vi "Test Master API.vi"() -> ()   [LabVIEW 2021, in "Master.lvlib"]
doc: "Master API Tester.\n\n<b>Note:</b> This VI was modified by the <b>Validate DQMH Module</b> tool to remove code to stop the main loop on error, and instead display the most recent error on the tester front panel."
uses:
  Master.lvlib
  <vilib>/Utility/error.llb/DialogType.ctl
panel:
  out "last error":errorcluster
  in  "SlaveID":i32(ring)=-1 items=["All"=-1, "1"=1, "2"=2, "3"=3, "4"=4, "5"=5, "6"=6, "7"=7, "8"=8, "9"=9, "10"=10, "11"=11, "12"=12, "13"=13, "14"=14, "15"=15, "16"=16, "17"=17, "18"=18, "19"=19, "20"=20, "21"=21, "22"=22, "23"=23, "24"=24, "25"=25, "26"=26, "27"=27, "28"=28, "29"=29, "30"=30, "31"=31, "32"=32, "33"=33, "34"=34, "35"=35, "36"=36, "37"=37, "38"=38, "39"=39, "40"=40, "41"=41, "42"=42, "43"=43, "44"=44, "45"=45, "46"=46, "47"=47, "48"=48, "49"=49, "50"=50, "51"=51, "52"=52, "53"=53, "54"=54, "55"=55, "56"=56, "57"=57, "58"=58, "59"=59, "60"=60, "61"=61, "62"=62, "63"=63, "64"=64, "65"=65, "66"=66, "67"=67, "68"=68, "69"=69, "70"=70, "71"=71, "72"=72, "73"=73, "74"=74, "75"=75, "76"=76, "77"=77, "78"=78, "79"=79, "80"=80, "81"=81, "82"=82, "83"=83, "84"=84, "85"=85, "86"=86, "87"=87, "88"=88, "89"=89, "90"=90, "91"=91, "92"=92, "93"=93, "94"=94, "95"=95, "96"=96, "97"=97, "98"=98, "99"=99, "100"=100, "101"=101, "102"=102, "103"=103, "104"=104, "105"=105, "106"=106, "107"=107, "108"=108, "109"=109, "110"=110, "111"=111, "112"=112, "113"=113, "114"=114, "115"=115, "116"=116, "117"=117, "118"=118, "119"=119, "120"=120, "121"=121, "122"=122, "123"=123, "124"=124, "125"=125, "126"=126, "127"=127, "128"=128, "129"=129, "130"=130, "131"=131, "132"=132, "133"=133, "134"=134, "135"=135, "136"=136, "137"=137, "138"=138, "139"=139, "140"=140, "141"=141, "142"=142, "143"=143, "144"=144, "145"=145, "146"=146, "147"=147, "148"=148, "149"=149, "150"=150, "151"=151, "152"=152, "153"=153, "154"=154, "155"=155, "156"=156, "157"=157, "158"=158, "159"=159, "160"=160, "161"=161, "162"=162, "163"=163, "164"=164, "165"=165, "166"=166, "167"=167, "168"=168, "169"=169, "170"=170, "171"=171, "172"=172, "173"=173, "174"=174, "175"=175, "176"=176, "177"=177, "178"=178, "179"=179, "180"=180, "181"=181, "182"=182]
  in  "Slave Stop":bool
  in  "Slave Launch":bool
  out "Title":string
  in  "Show Diagram on Init":bool
  in  "Show Block Diagram":bool
  in  "Stop Module":bool
  in  "Start Module":bool
  in  "Hide Module Panel":bool
  in  "Show Module Panel":bool
  out "Status":string
  out "Module Running?":bool
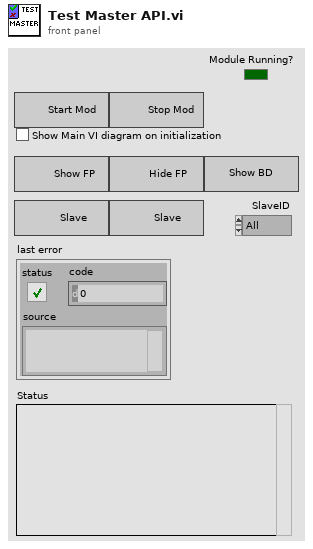
[diagram p1: front panel]
types:
  T1 = typedef "Master.lvlib/Broadcast Events--cluster.ctl" = cluster{"Module Did Init":refnum<user-event>, "Status Updated":refnum<user-event>, "Error Reported":refnum<user-event>, "Module Did Stop":refnum<user-event>, "Update Module Execution Status":refnum<user-event>, "Slave Launched":refnum<user-event>}
  T2 = typedef "DialogType.ctl" = u16
  T3 = typedef "LVStringsAndValuesArrayTypeDef_I32.ctl" = cluster{"String":string, "Value":i32}[]
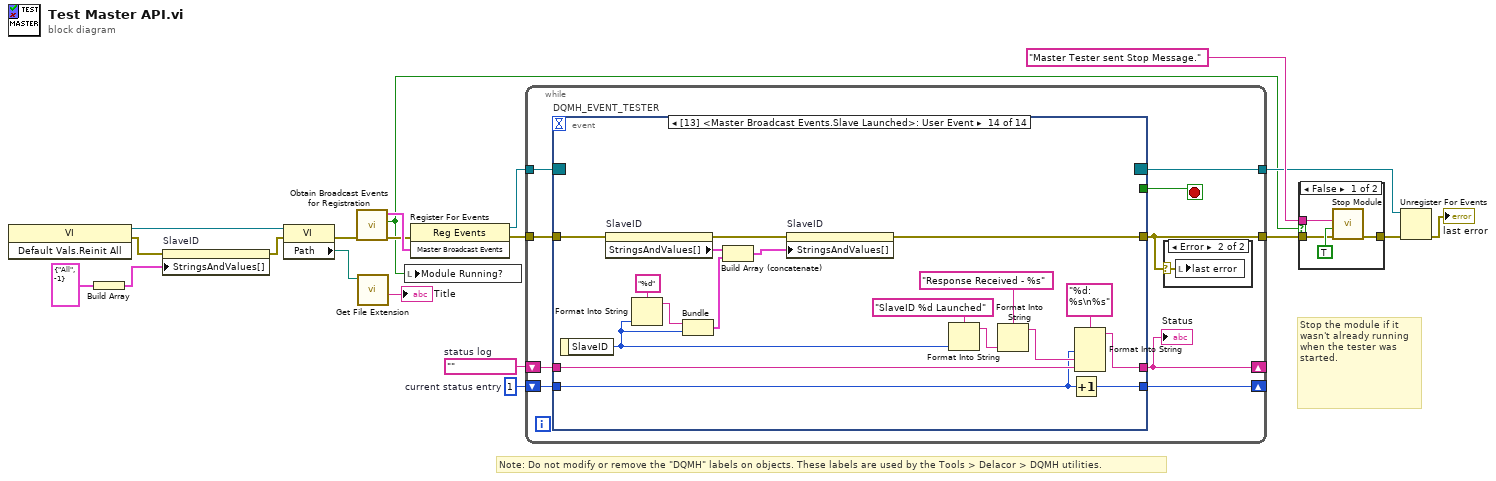
[diagram p0: block diagram]
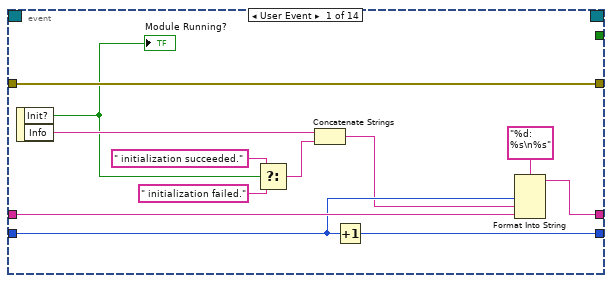
[diagram p4: hidden frame]
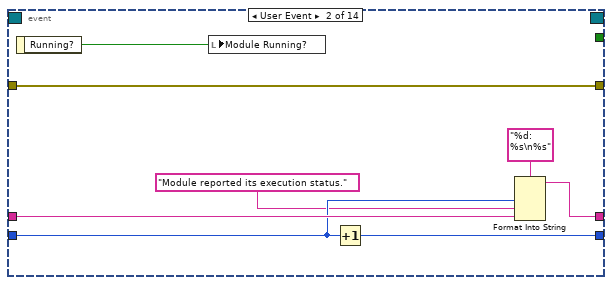
[diagram p5: hidden frame]
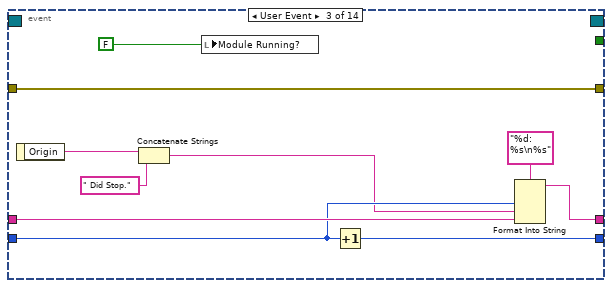
[diagram p6: hidden frame]
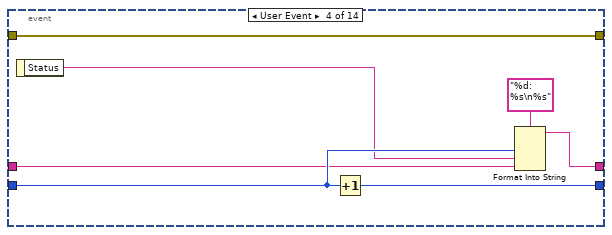
[diagram p7: hidden frame]
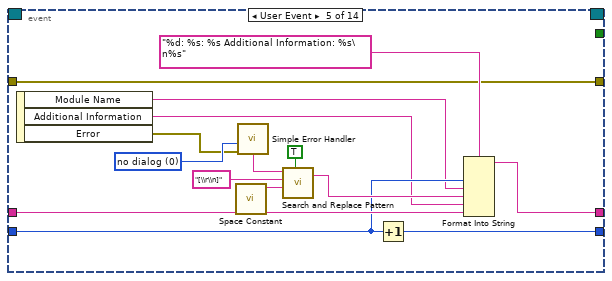
[diagram p8: hidden frame]
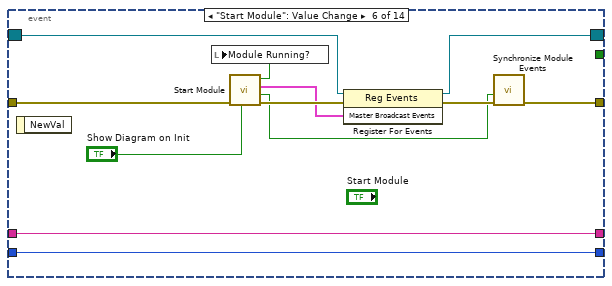
[diagram p9: hidden frame]
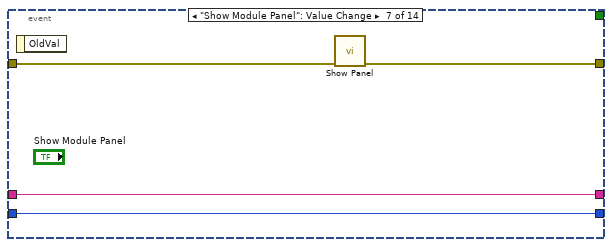
[diagram p10: hidden frame]
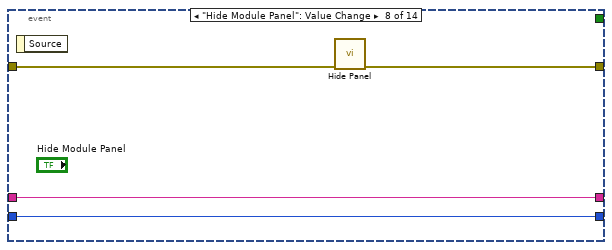
[diagram p11: hidden frame]
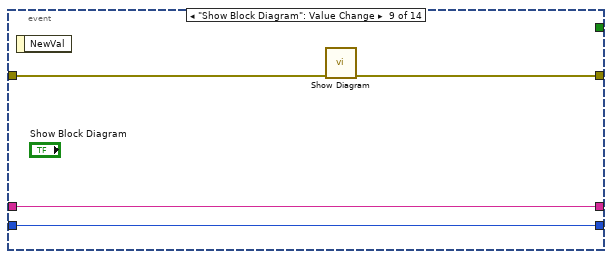
[diagram p12: hidden frame]
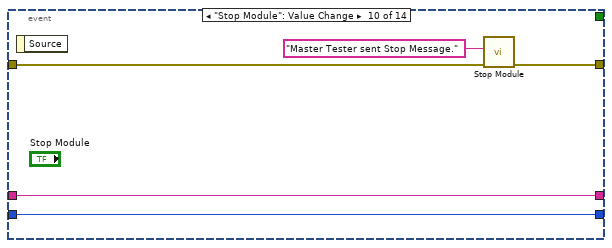
[diagram p13: hidden frame]
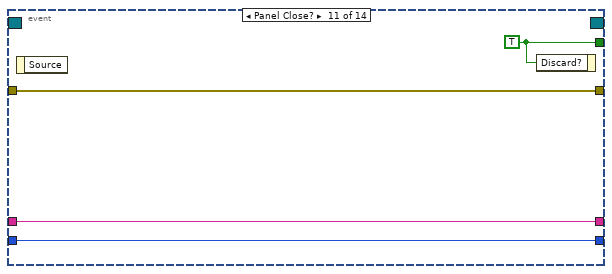
[diagram p14: hidden frame]
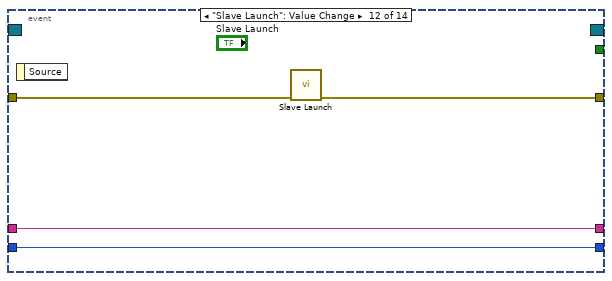
[diagram p15: hidden frame]
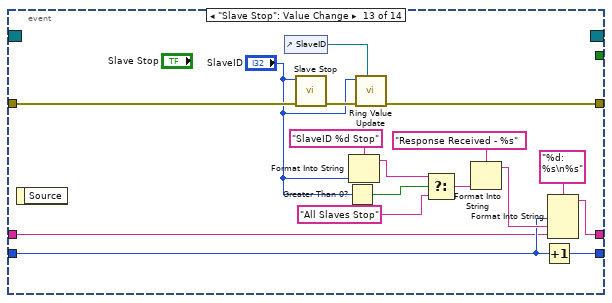
[diagram p16: hidden frame]
diagram:
  w17 = 1  # current status entry
  w18 = ""  # status log
  # "Stop the module if it wasn't already running when the tester was started."
  # "Note: Do not modify or remove the \"DQMH\" labels on objects. These labels are used by the Tools > Delacor > DQMH utilities."
  n1 = invoke class="VI" method="Default Vals.Reinit All"() -> (reference out=w9:refnum<vi>, error out=w5:errorcluster)  [unwired: 3 in, 1 out]
  n2 = Build Array(cluster{"String":string, "Value":i32} {"String"="All", "Value"=-1}) -> (w2:cluster{"String":string, "Value":i32}[])
  n3 = property on="SlaveID" class="Ring (strict)"(error in=w5, "StringsAndValues[]"=w2) -> (error out=w4:errorcluster)  [unwired: 1 in, 1 out]
  n4 = property class="VI"(reference=w9, error in=w4) -> (error out=w8:errorcluster, "Path"=w7:path)  [unwired: 1 out]
  n5 = call "Obtain Broadcast Events for Registration.vi"("error in"=w8) -> ("error out"=w12:errorcluster, "Already running?"=w11:bool, "Master Broadcast Events"=w15:T1)  [unwired: 8 in]
  n6 = call <vilib>:"Get File Extension.vi"("file"=w7) -> ("filename without extension"=→"Title":string)  [unwired: 6 in, 4 out]
  n7 = local write "Module Running?"(w11) -> ()
  n8 = register-events(error in=w12, w15) -> (reference out=w14:refnum<event-registration>, error out=w16:errorcluster)  [unwired: 1 in]
  n9 = while {
    tunnel: w14 -> [w29]
    tunnel: [w22] -> w10
    shift-right: [w25] -> _
    shift-left: w18 -> [w27]
    shift-right: [w26] -> _
    shift-left: w17 -> [w28]
    tunnel: w16 -> [w24]
    tunnel: [w23] -> w13
    stop <- w21 stop-if-true
    n10 = event "DQMH_EVENT_TESTER" shown="[13] <Master Broadcast Events.Slave Launched>: User Event" {
      selector: w29 -> [_ _ _ _ _ w88 _ _ _ _ _ _ _ _]
      dyn-events: [_ _ _ _ _ w87 _ _ _ _ _ _ _ _] -> w23
      timeout: _ -> [_ _ _ _ _ _ _ _ _ _ _ _ _ _]
      tunnel: [_ _ _ _ _ _ _ _ _ _ w115 _ _ _] -> w21
      tunnel: [w42 w44 w51 w61 w71 w86 w98 w102 w103 w109 w112 w116 w134 w147] -> w22
      tunnel: w28 -> [w39 w48 w58 w64 w74 w91 w96 w100 w104 w110 w113 w117 w129 w140]
      tunnel: w27 -> [w40 w49 w59 w63 w75 w92 w97 w101 w105 w111 w114 w118 w128 w141]
      tunnel: [w37 w46 w56 w65 w73 w92 w97 w101 w105 w111 w114 w118 w127 w139] -> w25
      tunnel: [w38 w47 w57 w67 w72 w91 w96 w100 w104 w110 w113 w117 w126 w138] -> w26
      tunnel: w24 -> [w42 w44 w51 w61 w71 w85 w95 w99 w106 w107 w112 w119 w136 w154]
      event User Event {
        n11 = event-data() -> ("Init?"=w34:bool, "Info"=w36:string)  [unwired: 1 in]
        "Module Running?" <- w34
        n12 = Select(t=" initialization succeeded.", s=w34, f=" initialization failed.") -> (s? t:f=w31:string)
        n13 = Concatenate Strings(w36, w31) -> (w35:string)
        n14 = Increment(x=w39) -> (x+1=w38:i32)
        n15 = Format Into String(format string="%d: %s\n%s", w39, w35, w40) -> (resulting string=w37:string)  [unwired: 2 in, 1 out]
      }
      event User Event {
        n16 = event-data() -> ("Running?"=w43:bool)  [unwired: 1 in]
        n17 = local write "Module Running?"(w43) -> ()
        n18 = Increment(x=w48) -> (x+1=w47:i32)
        n19 = Format Into String(format string="%d: %s\n%s", w48, "Module reported its execution status.", w49) -> (resulting string=w46:string)  [unwired: 2 in, 1 out]
      }
      event User Event {
        n20 = event-data() -> ("Origin"=w55:string)  [unwired: 1 in]
        n21 = Concatenate Strings(w55, " Did Stop.") -> (w54:string)
        n22 = local write "Module Running?"(FALSE ("Module Did Init?")) -> ()
        n23 = Increment(x=w58) -> (x+1=w57:i32)
        n24 = Format Into String(format string="%d: %s\n%s", w58, w54, w59) -> (resulting string=w56:string)  [unwired: 2 in, 1 out]
      }
      event User Event {
        n25 = event-data() -> ("Status"=w62:string)  [unwired: 1 in]
        n26 = Increment(x=w64) -> (x+1=w67:i32)
        n27 = Format Into String(format string="%d: %s\n%s", w64, w62, w63) -> (resulting string=w65:string)  [unwired: 2 in, 1 out]
      }
      event User Event {
        w76 = T2 0 items=["no dialog", "OK message", "continue or stop message", "OK message + warnings", "continue/stop + warnings"] ("type of dialog (OK msg:1)")
        n28 = event-data() -> ("Module Name"=w70:string, "Additional Information"=w69:string, "Error"=w68:errorcluster)  [unwired: 1 in]
        n29 = call <vilib>:"Space Constant.vi"() -> ("String"=w80:string)
        n30 = call <vilib>:"Simple Error Handler.vi"("type of dialog (OK msg:1)"=w76, "error in (no error)"=w68) -> ("message"=w77:string)  [unwired: 3 in, 4 out]
        n31 = call <vilib>:"Search and Replace Pattern.vi"("string"=w77, "regular expression (\"\")"="[\\r\\n]" ("regular expression (\"\")"), "replace string (\"\")"=w80, "replace all? (F)"=TRUE ("replace all CR/LF with spaces")) -> ("result string"=w78:string)  [unwired: 1 in, 1 out]
        n32 = Increment(x=w74) -> (x+1=w72:i32)
        n33 = Format Into String(format string="%d: %s: %s Additional Information: %s\n%s", w74, w70, w78, w69, w75) -> (resulting string=w73:string)  [unwired: 2 in, 1 out]
      }
      event "Start Module": Value Change {
        n34 = event-data() -> ()  [unwired: 1 in, 1 out]
        n35 = call "Start Module.vi"("Show Main VI Diagram on Init (F)"="Show Diagram on Init", "error in"=w85) -> ("error out"=w93:errorcluster, "Wait for Event Sync?"=w90:bool, "Master Broadcast Events"=w89:T1, "Module Was Already Running?"=w84:bool)  [unwired: 6 in]
        n36 = local write "Module Running?"(w84) -> ()
        n37 = register-events(reference=w88, error in=w93, w89) -> (reference out=w87:refnum<event-registration>, error out=w94:errorcluster)
        n38 = call "Synchronize Module Events.vi"("error in"=w94, "Wait for Event Sync?"=w90) -> ("error out"=w86:errorcluster)  [unwired: 9 in]
      }
      event "Show Module Panel": Value Change {
        n39 = event-data() -> ()  [unwired: 1 in, 1 out]
        n40 = call "Show Panel.vi"("error in (no error)"=w95) -> ("error out"=w98:errorcluster)  [unwired: 10 in]
      }
      event "Hide Module Panel": Value Change {
        n41 = event-data() -> ()  [unwired: 1 in, 1 out]
        n42 = call "Hide Panel.vi"("error in (no error)"=w99) -> ("error out"=w102:errorcluster)  [unwired: 10 in]
      }
      event "Show Block Diagram": Value Change {
        n43 = event-data() -> ()  [unwired: 1 in, 1 out]
        n44 = call "Show Diagram.vi"("error in (no error)"=w106) -> ("error out"=w103:errorcluster)  [unwired: 10 in]
      }
      event "Stop Module": Value Change {
        n45 = event-data() -> ()  [unwired: 1 in, 1 out]
        n46 = call "Stop Module.vi"("error in"=w107, "Origin"="Master Tester sent Stop Message.") -> ("error out"=w109:errorcluster)  [unwired: 9 in]
      }
      event Panel Close? {
        w115 = TRUE ("Discard?")
        n47 = event-data() -> ()  [unwired: 1 in, 1 out]
        n48 = event-data("Discard?"=w115) -> ()  [unwired: 1 in, 1 out]
      }
      event "Slave Launch": Value Change {
        n49 = event-data() -> ()  [unwired: 1 in, 1 out]
        n50 = call "Slave Launch.vi"("error in"=w119) -> ("error out"=w116:errorcluster)  [unwired: 10 in]
      }
      event "Slave Stop": Value Change {
        n51 = event-data() -> ()  [unwired: 1 in, 1 out]
        n52 = control-ref of="SlaveID"() -> (w121:refnum<vi>)
        n53 = call "Slave Stop.vi"("error in"=w136, "Module ID"="SlaveID") -> ("error out"=w135:errorcluster)  [unwired: 9 in]
        n54 = Greater Than 0?(x="SlaveID") -> (x > 0?=w122:bool)
        n55 = Format Into String(format string="SlaveID %d Stop", "SlaveID") -> (resulting string=w125:string)  [unwired: 2 in, 1 out]
        n56 = call "Ring Value Update.vi"("Ring in"=w121, "error in (no error)"=w135, "SlaveID"="SlaveID") -> ("error out"=w134:errorcluster)  [unwired: 8 in]
        n57 = Select(t=w125, s=w122, f="All Slaves Stop" ("format string")) -> (s? t:f=w124:string)
        n58 = Format Into String(format string="Response Received - %s", w124) -> (resulting string=w131:string)  [unwired: 2 in, 1 out]
        n59 = Increment(x=w129) -> (x+1=w126:i32)
        n60 = Format Into String(format string="%d: %s\n%s", w129, w131, w128) -> (resulting string=w127:string)  [unwired: 2 in, 1 out]
      }
      event User Event {
        n61 = event-data() -> ("SlaveID"=w137:i32)  [unwired: 1 in]
        n62 = property on="SlaveID" class="Ring (strict)"(error in=w154) -> (error out=w148:errorcluster, "StringsAndValues[]"=w153:T3)  [unwired: 1 in, 1 out]
        n63 = Format Into String(format string="%d", w137) -> (resulting string=w151:string)  [unwired: 2 in, 1 out]
        n64 = Bundle(w151, "SlaveID"=w137) -> (w150:cluster{string, "SlaveID":i32})  [unwired: 1 in]
        n65 = Build Array (concatenate)(w153, w150) -> (w149:T3)
        n66 = property on="SlaveID" class="Ring (strict)"(error in=w148, "StringsAndValues[]"=w149) -> (error out=w147:errorcluster)  [unwired: 1 in, 1 out]
        n67 = Format Into String(format string="SlaveID %d Launched", w137) -> (resulting string=w142:string)  [unwired: 2 in, 1 out]
        n68 = Format Into String(format string="Response Received - %s", w142) -> (resulting string=w144:string)  [unwired: 2 in, 1 out]
        n69 = Increment(x=w140) -> (x+1=w138:i32)
        n70 = Format Into String(format string="%d: %s\n%s", w140, w144, w141) -> (resulting string=w139:string)  [unwired: 2 in, 1 out]
      }
    }
    "Status" <- w25
    n71 = case "DQMH_TESTER_ERROR_LOCAL" shown="Error" w22 {
      selector: w22 -> [_ w30]
      frame No Error {
      }
      frame Error {
        n72 = local write "last error"(w30) -> ()
      }
    }
  }
  n73 = case shown="False" w11 {
    tunnel: [w158 w159] -> w20
    tunnel: "Master Tester sent Stop Message." ("Origin") -> [w157 _]
    tunnel: w10 -> [w155 w159]
    frame False {
      n74 = call "Stop Module.vi"("error in"=w155, "Wait for Module to Stop? (F)"=TRUE ("Wait for Module to stop?"), "Origin"=w157) -> ("error out"=w158:errorcluster)  [unwired: 8 in]
    }
    frame True {
    }
  }
  n75 = Unregister For Events(event registration refnum=w13, error in=w20) -> (error out=→"last error":errorcluster)
